vi "GetErrorCreationType.vi"(8 "error in (no error)":errorcluster) -> (0 "error out":errorcluster, 1 "ErrorCreationType":refnum<class "ErrorCreationExecution.lvclass">)   [LabVIEW 2018, in "ErrorCreationExecution.lvclass"]
uses:
  <userlib>/_express/CustomErrorCreator/ErrorCreationExecution/ErrorCreationExecution.lvclass
  <userlib>/_express/CustomErrorCreator/ErrorCreationExecution/ErrorCreationType.vi
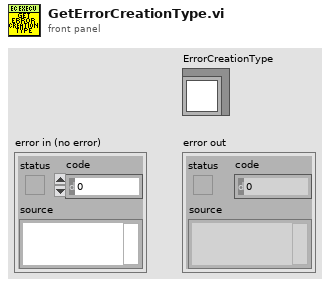
[diagram p1: front panel]
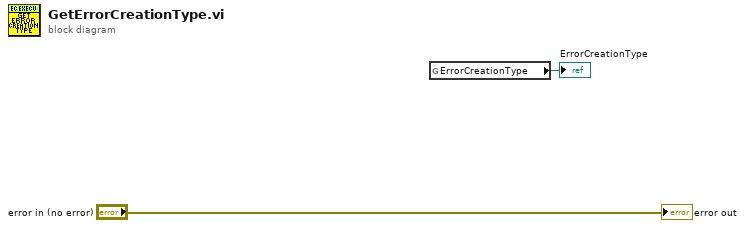
[diagram p0: block diagram]
diagram:
  n1 = global read "ErrorCreationType.vi" "ErrorCreationType"() -> (→"ErrorCreationType":refnum<class "ErrorCreationExecution.lvclass">)
  "error out" <- "error in (no error)"
